vi "Recursive Data Structure for Control Properties.vi"(5 "Max Level (10)":i32, 6 "Draw Controls":T1={"Subpanels"=TRUE, "Tabs"=FALSE, "TypeDefs"=FALSE, "Error Clusters"=enum."Ignore", "DVRs"=enum."Ignore", "Queues & Notifiers"=enum."Ignore"}, 7 "Ignore Image Data (F)":bool, 8 "error in":errorcluster, 9 "Current Level (0)":i32, 10 "Controls[]":refnum<vi>[](array[refnum]), 11 "Parent's name":string) -> (0 "error out":errorcluster, 2 "Results":T3[](array[typedef]))   [LabVIEW 2023, in "VIDoc Parsing.lvlib"]
uses:
  VIDoc Parsing.lvlib
  TypeDefs/Controls Info Cluster.ctl
  <vilib>/picture/picture.llb/imagedata.ctl
  <vilib>/Utility/miscctls.llb/LVKeyTypeDef.ctl
  Settings/Parser Settings/Draw Controls Cluster.ctl
  Settings/Parser Settings/Draw Option Enum.ctl
  <vilib>/Utility/error.llb/Trim Whitespace One-Sided.vi
  Settings/Parser Settings/Parser Settings.lvclass
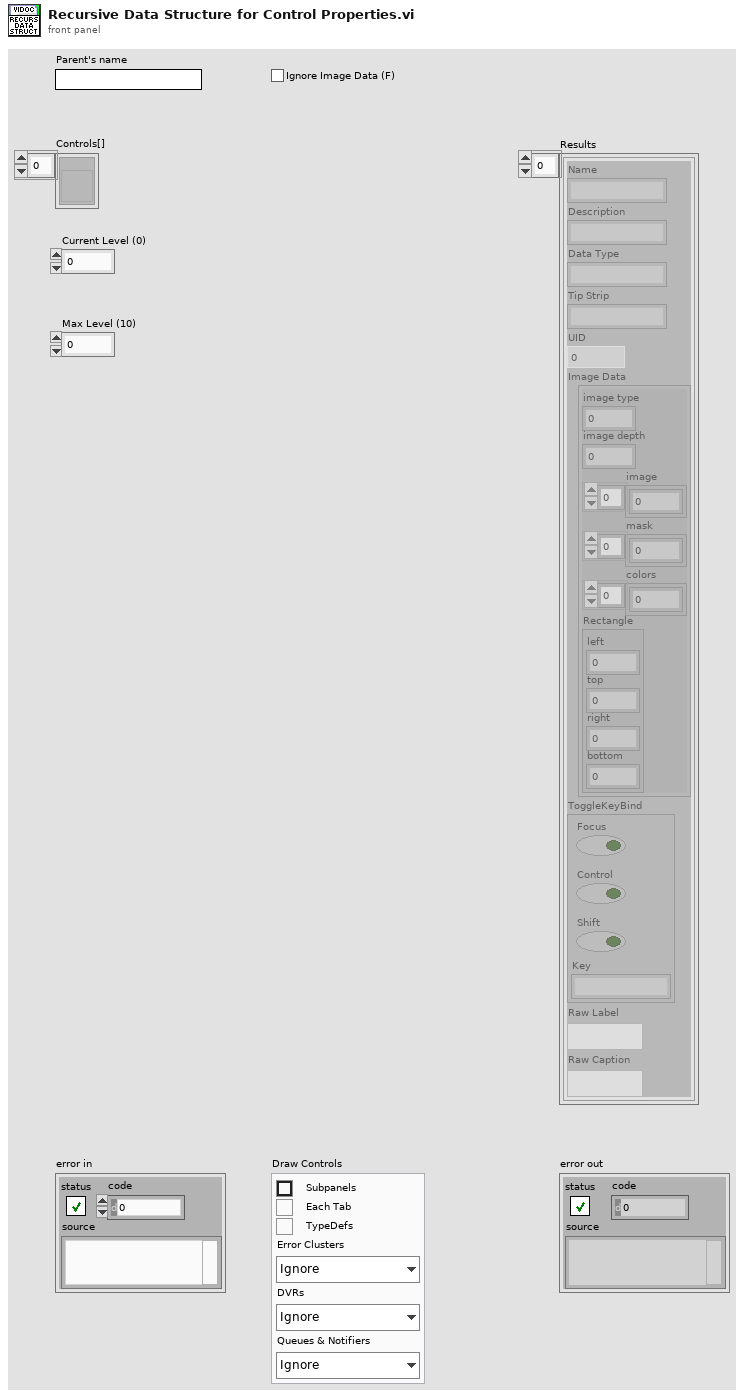
[diagram p1: front panel]
types:
  T1 = typedef "VIDoc Parsing.lvlib/Parser Settings.lvclass/Draw Controls Cluster.ctl" = cluster{"Subpanels":bool, "Tabs":bool, "TypeDefs":bool, "Error Clusters":T2, "DVRs":T2, "Queues & Notifiers":T2}
  T2 = typedef "VIDoc Parsing.lvlib/Parser Settings.lvclass/Draw Option Enum.ctl" = enum16{"Ignore", "Draw", "Draw + Contents"}
  T3 = typedef "VIDoc Parsing.lvlib/Controls Info Cluster.ctl" = cluster{"Name":string, "Description":string, "Data Type":string, "Tip Strip":string, "UID":i32, "Image Data":T4, "ToggleKeyBind":T5, "Raw Label":string, "Raw Caption":string}
  T4 = typedef "imagedata.ctl" = cluster{"image type":i32, "image depth":i32, "image":u8[], "mask":u8[], "colors":u32[], "Rectangle":cluster{"left":i16, "top":i16, "right":i16, "bottom":i16}}
  T5 = typedef "LVKeyTypeDef.ctl" = cluster{"Focus":bool, "Control":bool, "Shift":bool, "Key":string}
  T6 = enum32{"not a typedef", "typedef", "strict typedef", "class private data"}
  T7 = typedef "LVNumericRepresentation.ctl" = enum32{"Extended Precision", "Double Precision", "Single Precision", "Long", "Word", "Byte", "Unsigned Long", "Unsigned Word", "Unsigned Byte", "Complex Extended", "Complex Double", "Complex Single", "Quad", "Unsigned Quad", "Fixed-Point"}
  T8 = typedef "LVStringsAndValuesArrayTypeDef.ctl" = cluster{"String":string, "Value":ext}[]
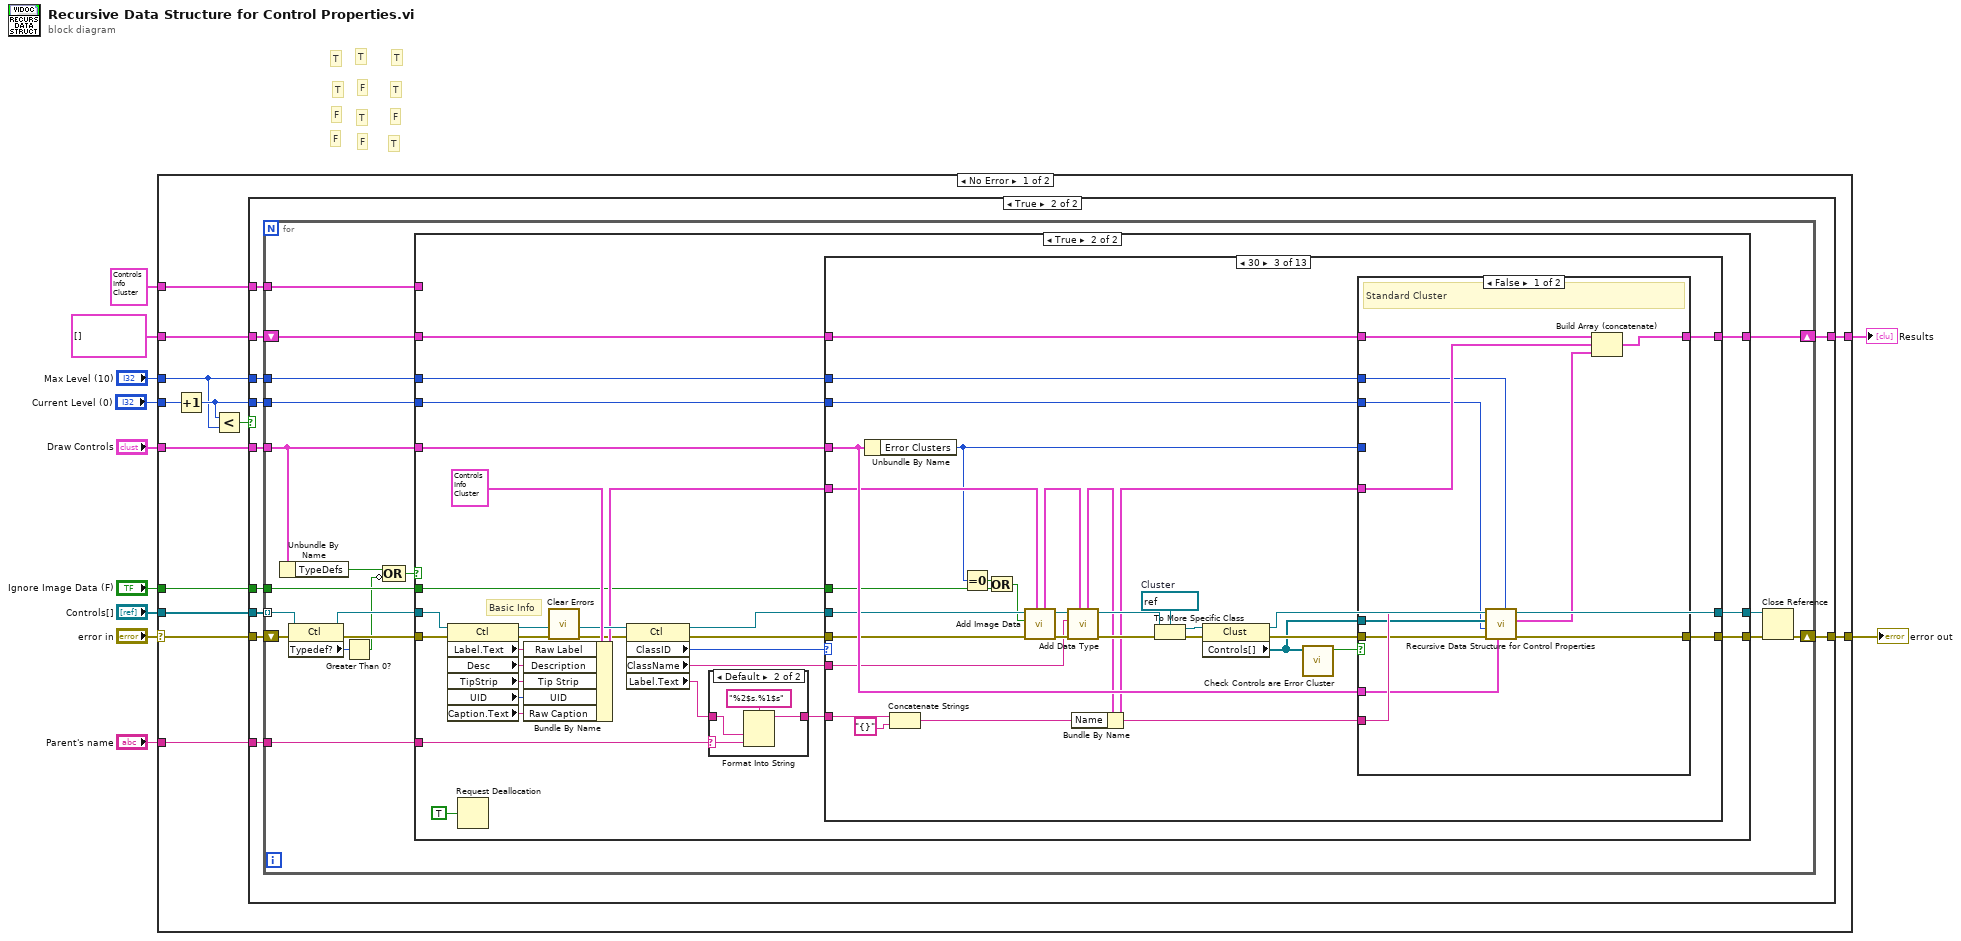
[diagram p0: block diagram]
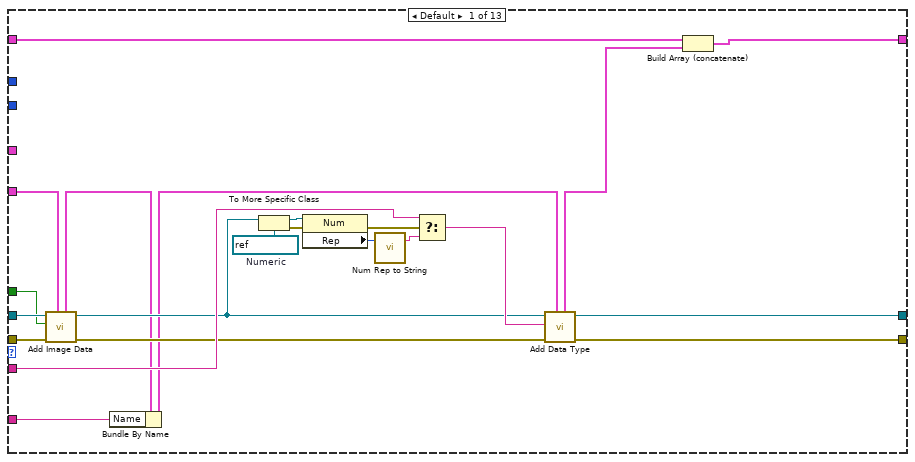
[diagram p5: hidden frame]
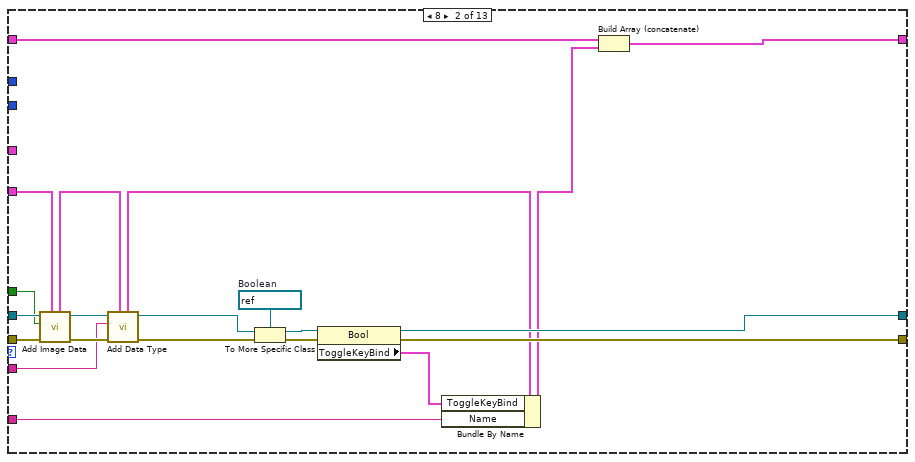
[diagram p6: hidden frame]
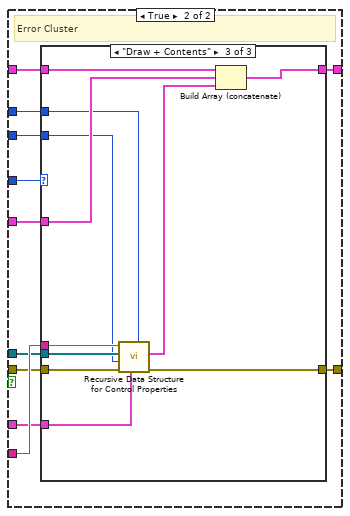
[diagram p7: hidden frame]
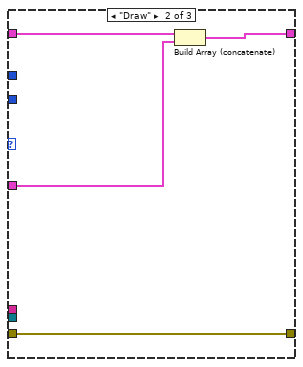
[diagram p9: hidden frame]
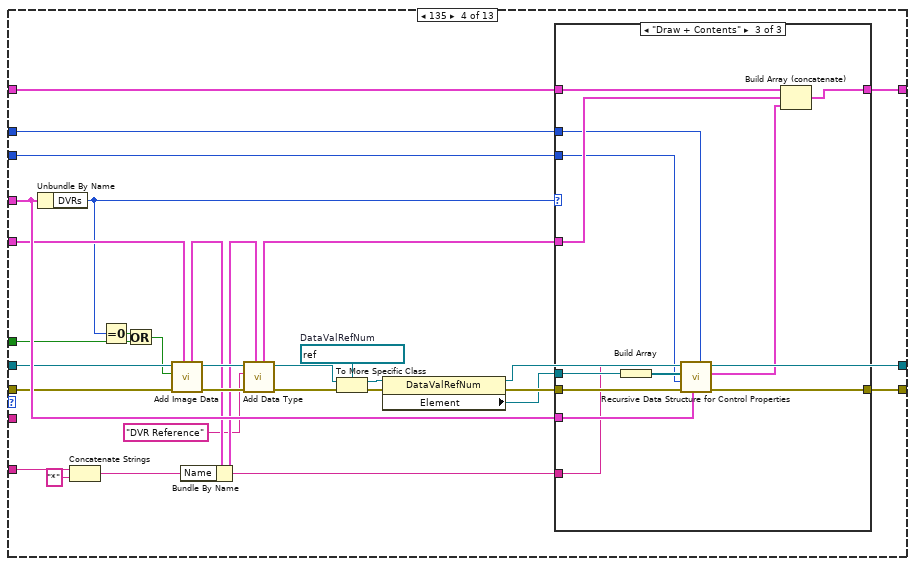
[diagram p10: hidden frame]
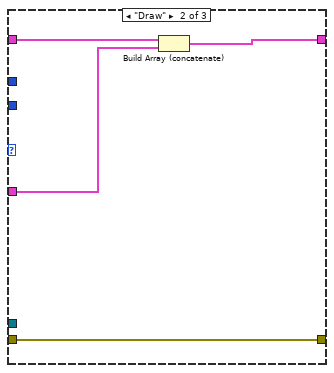
[diagram p12: hidden frame]
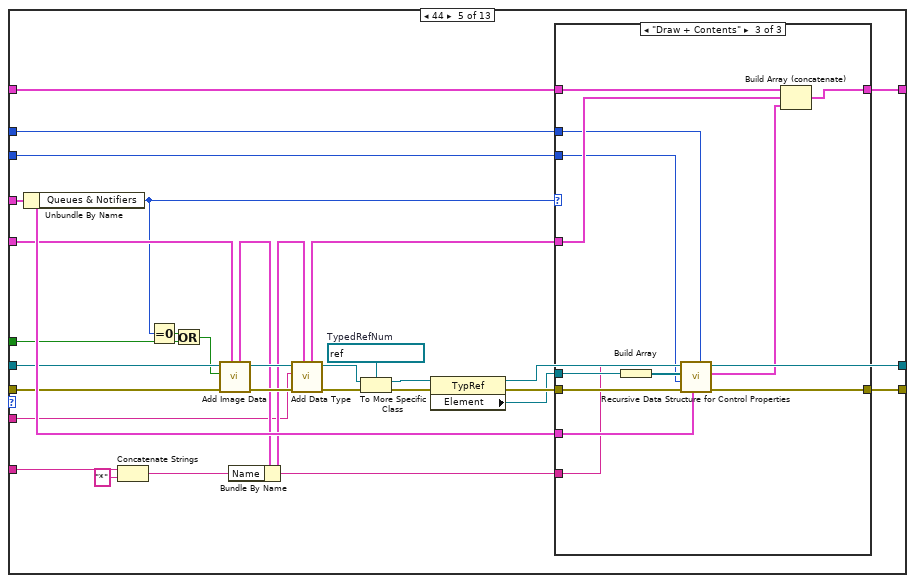
[diagram p13: hidden frame]
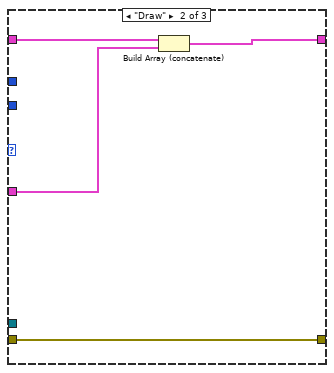
[diagram p15: hidden frame]
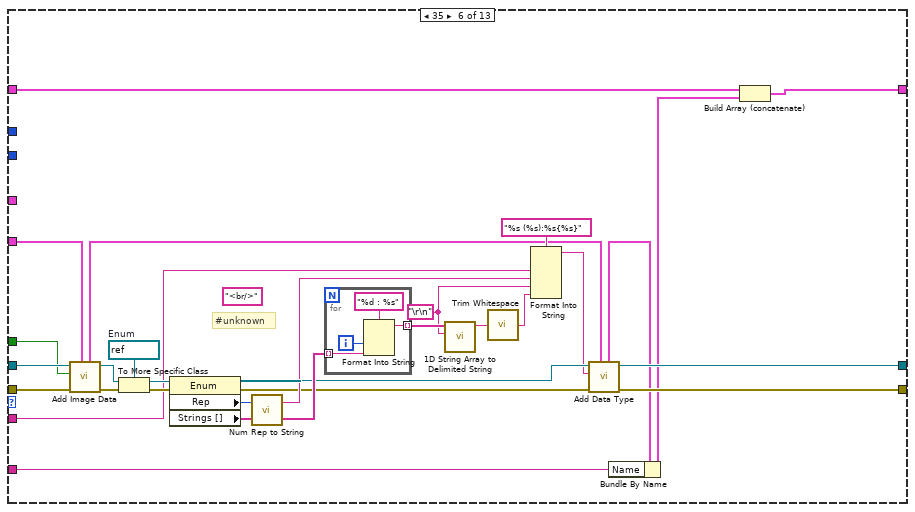
[diagram p16: hidden frame]
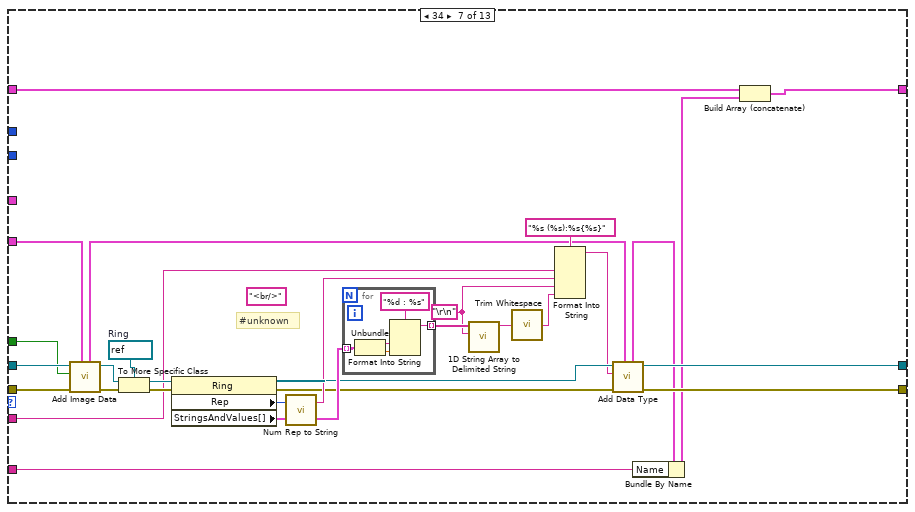
[diagram p17: hidden frame]
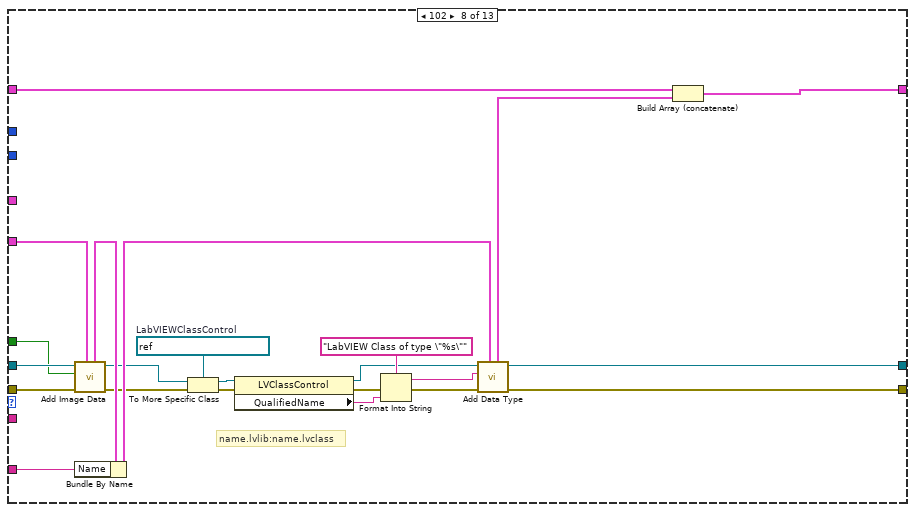
[diagram p18: hidden frame]
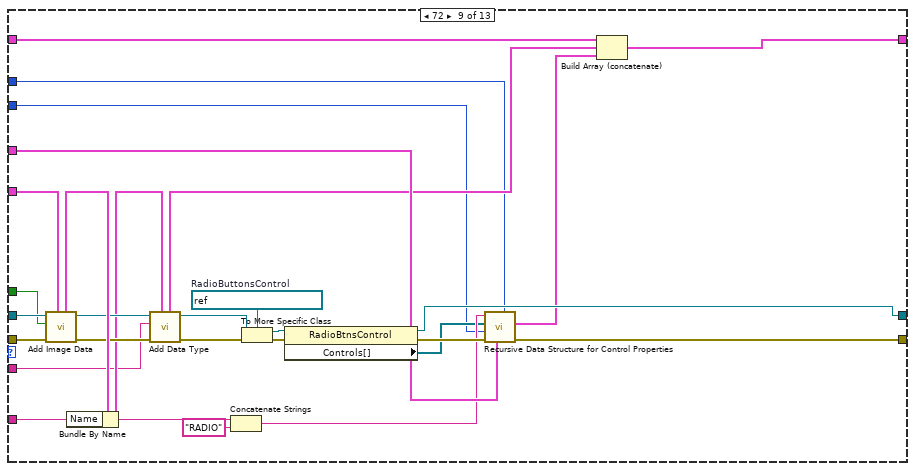
[diagram p19: hidden frame]
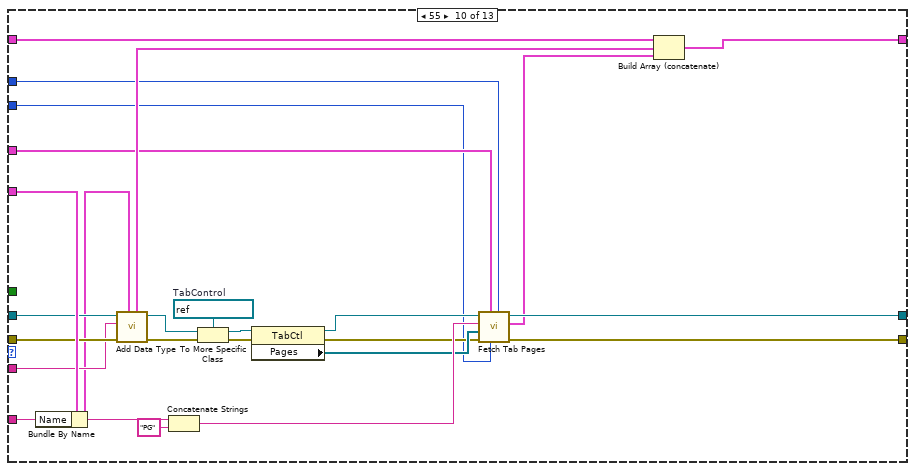
[diagram p20: hidden frame]
diagram:
  # "T"
  # "T"
  # "F"
  # "T"
  # "T"
  # "T"
  # "F"
  # "F"
  # "F"
  # "F"
  # "T"
  # "T"
  n1 = case shown="No Error" "error in" {
    selector: "error in" -> [w20 w517]
    tunnel: "Parent's name" -> [w22 _]
    tunnel: "Controls[]" -> [w24 _]
    tunnel: [w23 w517] -> w9
    tunnel: T3 {"Name"="", "Description"="", "Data Type"="", "Tip Strip"="", "UID"=0, "Image Data"={"image type"=0, "image depth"=0, "image"=[], "mask"=[], "colors"=[], "Rectangle"={"left"=0, "top"=0, "right"=0, "bottom"=0}}, "ToggleKeyBind"={"Focus"=FALSE, "Control"=FALSE, "Shift"=FALSE, "Key"=""}, "Raw Label"="", "Raw Caption"=""} -> [w21 _]
    tunnel: "Draw Controls" -> [w19 _]
    tunnel: "Ignore Image Data (F)" -> [w18 _]
    tunnel: T3[] [] -> [w17 w516]
    tunnel: [w16 w516] -> w3
    tunnel: "Current Level (0)" -> [w15 _]
    tunnel: "Max Level (10)" -> [w13 _]
    frame No Error {
      n2 = Increment(x=w15) -> (x+1=w14:i32)
      n3 = Less?(x=w14, y=w13) -> (x < y?=w12:bool)
      n4 = case shown="True" w12 {
        tunnel: w24 -> [_ w37]
        tunnel: [w25 w36] -> w23
        tunnel: w22 -> [_ w35]
        tunnel: w21 -> [_ w34]
        tunnel: w20 -> [w25 w33]
        tunnel: w19 -> [_ w32]
        tunnel: w18 -> [_ w31]
        tunnel: w17 -> [w26 w30]
        tunnel: [w26 w29] -> w16
        tunnel: w14 -> [_ w28]
        tunnel: w13 -> [_ w27]
        frame False {
        }
        frame True {
          n5 = for {
            tunnel: w37 -> [w48] mode=indexing
            tunnel: w35 -> [w56]
            tunnel: w34 -> [w55]
            shift-right: [w44] -> w36
            shift-left: w33 -> [w51]
            tunnel: w32 -> [w54]
            tunnel: w31 -> [w53]
            shift-right: [w46] -> w29
            shift-left: w30 -> [w52]
            tunnel: w28 -> [w39]
            tunnel: w27 -> [w38]
            n6 = Unbundle By Name(w54) -> ("TypeDefs"=w42:bool)
            n7 = property class="Ctl"(reference=w48, error in=w51) -> (reference out=w49:refnum<vi>, error out=w50:errorcluster, "Typedef?"=w47:T6)
            n8 = Greater Than 0?(x=w47) -> (x > 0?=w41:bool)
            n9 = Compound Arithmetic op=OR(w42, invert w41) -> (w40:bool)
            n10 = case shown="True" w40 {
              tunnel: w56 -> [_ w87]
              tunnel: w55 -> [_ _]
              tunnel: [w58 w64] -> w45
              tunnel: w54 -> [_ w79]
              tunnel: w53 -> [_ w69]
              tunnel: w52 -> [w59 w68]
              tunnel: w50 -> [w58 w67]
              tunnel: w49 -> [w57 w66]
              tunnel: [w59 w63] -> w46
              tunnel: [w57 w65] -> w43
              tunnel: w39 -> [_ w61]
              tunnel: w38 -> [_ w60]
              frame False {
                # "Is TypeDef but options say not to process"
              }
              frame True {
                # "Basic Info"
                n11 = property class="Ctl"(reference=w66, error in=w67) -> (reference out=w71:refnum<vi>, error out=w72:errorcluster, "Label.Text"=w77:string, "Desc"=w76:string, "TipStrip"=w75:string, "UID"=w74:i32, "Caption.Text"=w73:string)
                n12 = Request Deallocation(TRUE ("flag")) -> ()
                n13 = Bundle By Name(cluster=T3 {"Name"="", "Description"="", "Data Type"="", "Tip Strip"="", "UID"=0, "Image Data"={"image type"=0, "image depth"=0, "image"=[], "mask"=[], "colors"=[], "Rectangle"={"left"=0, "top"=0, "right"=0, "bottom"=0}}, "ToggleKeyBind"={"Focus"=FALSE, "Control"=FALSE, "Shift"=FALSE, "Key"=""}, "Raw Label"="", "Raw Caption"=""}, "Raw Label"=w77, "Description"=w76, "Tip Strip"=w75, "UID"=w74, "Raw Caption"=w73) -> (w70:T3)
                n14 = call <vilib>:"Clear Errors.vi"("error in (no error)"=w72) -> ("error out"=w62:errorcluster)  [unwired: 5 in, 1 out]
                n15 = property class="Ctl"(reference=w71, error in=w62) -> (reference out=w81:refnum<vi>, error out=w80:errorcluster, "ClassID"=w84:u32, "ClassName"=w85:string, "Label.Text"=w83:string)
                n16 = case shown="Default" w87 {
                  selector: w87 -> [_ w90]
                  tunnel: w83 -> [w88 w91]
                  tunnel: [w88 w89] -> w86
                  frame "" {
                  }
                  frame Default {
                    n17 = Format Into String(format string="%2$s.%1$s", w91, w90) -> (resulting string=w89:string)  [unwired: 2 in, 1 out]
                  }
                }
                n18 = case shown="30" w84 {
                  tunnel: w81 -> [w106 w130 w154 w225 w274 w322 w355 w385 w414 w437 w461 w487 w514]
                  tunnel: [w100 w131 w164 w229 w278 w308 w341 w370 w401 w424 w449 w477 w504] -> w64
                  tunnel: w86 -> [w105 w126 w161 w234 w282 w303 w336 w380 w409 w439 w456 w493 w507]
                  tunnel: [w98 w132 w160 w228 w277 w307 w340 w373 w415 w428 w451 w479 w498] -> w65
                  tunnel: w85 -> [w109 w120 w146 _ w256 w325 w358 _ w404 w435 _ w490 w503]
                  tunnel: w80 -> [w107 w129 w155 w224 w273 w321 w354 w384 w413 w436 w460 w486 w513]
                  tunnel: w79 -> [_ _ w158 w226 w275 _ _ _ w400 w423 _ w476 w515]
                  tunnel: w70 -> [w104 w127 w153 w223 w272 w319 w352 w382 w411 w440 w458 w484 w509]
                  tunnel: w69 -> [w103 w128 w139 w208 w258 w320 w353 w383 w412 _ w459 w485 w512]
                  tunnel: w68 -> [w95 w125 w142 w211 w261 w315 w348 w378 w397 w432 w447 w471 w501]
                  tunnel: [w94 w124 w141 w209 w259 w314 w347 w377 w396 w431 w446 w470 w500] -> w63
                  tunnel: w61 -> [_ _ w136 w206 w255 _ _ _ w392 w420 _ w466 _]
                  tunnel: w60 -> [_ _ w137 w207 w254 _ _ _ w393 w421 _ w467 _]
                  frame Default {
                    w111 = refnum<vi> refnum  # Numeric
                    n19 = call "Add Image Data.vi"("Control Info Cluster in"=w104, "error in (no error)"=w107, "Ignore Image Data"=w103, "Control in"=w106) -> ("error out"=w101:errorcluster, "Control out"=w99:refnum<vi>, "Control Info Cluster out"=w97:T3)  [unwired: 5 in]
                    n20 = Bundle By Name(cluster=w97, "Name"=w105) -> (w96:T3)
                    n21 = To More Specific Class(target class=w111, reference=w99) -> (specific class reference=w112:refnum<vi>, error out=w113:errorcluster)  [unwired: 1 in]
                    n22 = property class="Num"(reference=w112, error in=w113) -> (error out=w110:errorcluster, "Rep"=w114:T7)  [unwired: 1 out]
                    n23 = call "Num Rep to String.vi"("Rep"=w114) -> ("String"=w108:string)  [unwired: 2 in]
                    n24 = Select(t=w109, s=w110, f=w108) -> (s? t:f=w102:string)
                    n25 = call "Add Data Type.vi"("Control Info Cluster in"=w96, "error in (no error)"=w101, "Data Type String"=w102, "Control in"=w99) -> ("error out"=w100:errorcluster, "Control out"=w98:refnum<vi>, "Control Info Cluster out"=w93:T3)  [unwired: 4 in, 1 out]
                    n26 = Build Array (concatenate)(w95, w93) -> (w94:T3[])
                  }
                  frame 8 {
                    w135 = refnum<vi> refnum  # Boolean
                    n27 = call "Add Image Data.vi"("Control Info Cluster in"=w127, "error in (no error)"=w129, "Ignore Image Data"=w128, "Control in"=w130) -> ("error out"=w121:errorcluster, "Control out"=w123:refnum<vi>, "Control Info Cluster out"=w117:T3)  [unwired: 5 in]
                    n28 = call "Add Data Type.vi"("Control Info Cluster in"=w117, "error in (no error)"=w121, "Data Type String"=w120, "Control in"=w123) -> ("error out"=w118:errorcluster, "Control out"=w122:refnum<vi>, "Control Info Cluster out"=w116:T3)  [unwired: 4 in, 1 out]
                    n29 = To More Specific Class(target class=w135, reference=w122, error in=w118) -> (specific class reference=w134:refnum<vi>, error out=w133:errorcluster)
                    n30 = property class="Bool"(reference=w134, error in=w133) -> (reference out=w132:refnum<vi>, error out=w131:errorcluster, "ToggleKeyBind"=w119:T5)
                    n31 = Bundle By Name(cluster=w116, "ToggleKeyBind"=w119, "Name"=w126) -> (w115:T3)
                    n32 = Build Array (concatenate)(w125, w115) -> (w124:T3[])
                  }
                  frame 30 {
                    w166 = refnum<vi> refnum  # Cluster
                    n33 = Unbundle By Name(w158) -> ("Error Clusters"=w152:T2)
                    n34 = Concatenate Strings(w161, "{}" ("string")) -> (w143:string)
                    n35 = Equal To 0?(x=w152) -> (x = 0?=w151:bool)
                    n36 = Or(x=w151, y=w139) -> (x .or. y?=w140:bool)
                    n37 = call "Add Image Data.vi"("Control Info Cluster in"=w153, "error in (no error)"=w155, "Ignore Image Data"=w140, "Control in"=w154) -> ("error out"=w150:errorcluster, "Control out"=w148:refnum<vi>, "Control Info Cluster out"=w145:T3)  [unwired: 5 in]
                    n38 = call "Add Data Type.vi"("Control Info Cluster in"=w145, "error in (no error)"=w150, "Data Type String"=w146, "Control in"=w148) -> ("error out"=w149:errorcluster, "Control out"=w147:refnum<vi>, "Control Info Cluster out"=w144:T3)  [unwired: 4 in, 1 out]
                    n39 = Bundle By Name(cluster=w144, "Name"=w143) -> (w138:T3)
                    n40 = To More Specific Class(target class=w166, reference=w147, error in=w149) -> (specific class reference=w165:refnum<vi>, error out=w163:errorcluster)
                    n41 = property class="Clust"(reference=w165, error in=w163) -> (reference out=w160:refnum<vi>, error out=w159:errorcluster, "Controls[]"=w157:refnum<vi>[])
                    n42 = call "Check Controls are Error Cluster.vi"("Controls[]"=w157) -> ("Error Cluster"=w156:bool)  [unwired: 10 in]
                    n43 = case shown="False" w156 {
                      tunnel: [w174 w188] -> w164
                      tunnel: w143 -> [w177 w187]
                      tunnel: w157 -> [w173 w186]
                      tunnel: w159 -> [w176 w185]
                      tunnel: w158 -> [w175 w184]
                      tunnel: w152 -> [_ w183]
                      tunnel: w142 -> [w172 w180]
                      tunnel: [w171 w181] -> w141
                      tunnel: w138 -> [w169 w182]
                      tunnel: w137 -> [w168 w179]
                      tunnel: w136 -> [w167 w178]
                      frame False {
                        # "Standard Cluster"
                        n44 = call "Recursive Data Structure for Control Properties.vi"("Max Level (10)"=w168, "Draw Controls"=w175, "error in"=w176, "Current Level (0)"=w167, "Controls[]"=w173, "Parent's name"=w177) -> ("error out"=w174:errorcluster, "Results"=w170:T3[])  [unwired: 4 in]
                        n45 = Build Array (concatenate)(w172, w169, w170) -> (w171:T3[])
                      }
                      frame True {
                        # "Error Cluster"
                        n46 = case shown="\"Draw + Contents\"" w183 {
                          tunnel: w186 -> [_ _ w201]
                          tunnel: [w190 w194 w204] -> w188
                          tunnel: w187 -> [_ _ w202]
                          tunnel: w185 -> [w190 w194 w205]
                          tunnel: w184 -> [_ _ w203]
                          tunnel: w182 -> [_ w191 w198]
                          tunnel: [w189 w192 w199] -> w181
                          tunnel: w180 -> [w189 w193 w200]
                          tunnel: w179 -> [_ _ w196]
                          tunnel: w178 -> [_ _ w195]
                          frame "Ignore" {
                          }
                          frame "Draw" {
                            n47 = Build Array (concatenate)(w193, w191) -> (w192:T3[])
                          }
                          frame "Draw + Contents" {
                            n48 = call "Recursive Data Structure for Control Properties.vi"("Max Level (10)"=w196, "Draw Controls"=w203, "error in"=w205, "Current Level (0)"=w195, "Controls[]"=w201, "Parent's name"=w202) -> ("error out"=w204:errorcluster, "Results"=w197:T3[])  [unwired: 4 in]
                            n49 = Build Array (concatenate)(w200, w198, w197) -> (w199:T3[])
                          }
                        }
                      }
                    }
                  }
                  frame 135 {
                    w233 = refnum<vi> refnum  # DataValRefNum
                    n50 = Unbundle By Name(w226) -> ("DVRs"=w221:T2)
                    n51 = Concatenate Strings(w234, "*" ("string")) -> (w214:string)
                    n52 = Equal To 0?(x=w221) -> (x = 0?=w222:bool)
                    n53 = Or(x=w222, y=w208) -> (x .or. y?=w220:bool)
                    n54 = call "Add Image Data.vi"("Control Info Cluster in"=w223, "error in (no error)"=w224, "Ignore Image Data"=w220, "Control in"=w225) -> ("error out"=w218:errorcluster, "Control out"=w219:refnum<vi>, "Control Info Cluster out"=w215:T3)  [unwired: 5 in]
                    n55 = Bundle By Name(cluster=w215, "Name"=w214) -> (w213:T3)
                    n56 = call "Add Data Type.vi"("Control Info Cluster in"=w213, "error in (no error)"=w218, "Data Type String"="DVR Reference" ("input 2"), "Control in"=w219) -> ("error out"=w217:errorcluster, "Control out"=w216:refnum<vi>, "Control Info Cluster out"=w210:T3)  [unwired: 4 in, 1 out]
                    n57 = To More Specific Class(target class=w233, reference=w216, error in=w217) -> (specific class reference=w227:refnum<vi>, error out=w232:errorcluster)
                    n58 = property class="DataValRefNum"(reference=w227, error in=w232) -> (reference out=w228:refnum<vi>, error out=w231:errorcluster, "Element"=w230:refnum<vi>)
                    n59 = case shown="\"Draw + Contents\"" w221 {
                      tunnel: w214 -> [_ _ w246]
                      tunnel: w231 -> [w237 w241 w249]
                      tunnel: w230 -> [_ _ w253]
                      tunnel: [w237 w241 w248] -> w229
                      tunnel: w226 -> [_ _ w247]
                      tunnel: w211 -> [w236 w240 w252]
                      tunnel: w210 -> [_ w238 w250]
                      tunnel: [w236 w239 w251] -> w209
                      tunnel: w207 -> [_ _ w243]
                      tunnel: w206 -> [_ _ w242]
                      frame "Ignore" {
                      }
                      frame "Draw" {
                        n60 = Build Array (concatenate)(w240, w238) -> (w239:T3[])
                      }
                      frame "Draw + Contents" {
                        n61 = Build Array(w253) -> (w245:refnum<vi>[])
                        n62 = call "Recursive Data Structure for Control Properties.vi"("Max Level (10)"=w243, "Draw Controls"=w247, "error in"=w249, "Current Level (0)"=w242, "Controls[]"=w245, "Parent's name"=w246) -> ("error out"=w248:errorcluster, "Results"=w244:T3[])  [unwired: 4 in]
                        n63 = Build Array (concatenate)(w252, w250, w244) -> (w251:T3[])
                      }
                    }
                  }
                  frame 44 {
                    w257 = refnum<vi> refnum  # TypedRefNum
                    n64 = Unbundle By Name(w275) -> ("Queues & Notifiers"=w270:T2)
                    n65 = Concatenate Strings(w282, "*" ("string")) -> (w263:string)
                    n66 = Equal To 0?(x=w270) -> (x = 0?=w271:bool)
                    n67 = Or(x=w271, y=w258) -> (x .or. y?=w269:bool)
                    n68 = call "Add Image Data.vi"("Control Info Cluster in"=w272, "error in (no error)"=w273, "Ignore Image Data"=w269, "Control in"=w274) -> ("error out"=w267:errorcluster, "Control out"=w268:refnum<vi>, "Control Info Cluster out"=w264:T3)  [unwired: 5 in]
                    n69 = Bundle By Name(cluster=w264, "Name"=w263) -> (w262:T3)
                    n70 = call "Add Data Type.vi"("Control Info Cluster in"=w262, "error in (no error)"=w267, "Data Type String"=w256, "Control in"=w268) -> ("error out"=w266:errorcluster, "Control out"=w265:refnum<vi>, "Control Info Cluster out"=w260:T3)  [unwired: 4 in, 1 out]
                    n71 = To More Specific Class(target class=w257, reference=w265, error in=w266) -> (specific class reference=w276:refnum<vi>, error out=w281:errorcluster)
                    n72 = property class="TypRef"(reference=w276, error in=w281) -> (reference out=w277:refnum<vi>, error out=w280:errorcluster, "Element"=w279:refnum<vi>)
                    n73 = case shown="\"Draw + Contents\"" w270 {
                      tunnel: w263 -> [_ _ w294]
                      tunnel: w280 -> [w285 w289 w297]
                      tunnel: w279 -> [_ _ w301]
                      tunnel: [w285 w289 w296] -> w278
                      tunnel: w275 -> [_ _ w295]
                      tunnel: w261 -> [w284 w288 w300]
                      tunnel: w260 -> [_ w286 w298]
                      tunnel: [w284 w287 w299] -> w259
                      tunnel: w255 -> [_ _ w291]
                      tunnel: w254 -> [_ _ w290]
                      frame "Ignore" {
                      }
                      frame "Draw" {
                        n74 = Build Array (concatenate)(w288, w286) -> (w287:T3[])
                      }
                      frame "Draw + Contents" {
                        n75 = Build Array(w301) -> (w293:refnum<vi>[])
                        n76 = call "Recursive Data Structure for Control Properties.vi"("Max Level (10)"=w290, "Draw Controls"=w295, "error in"=w297, "Current Level (0)"=w291, "Controls[]"=w293, "Parent's name"=w294) -> ("error out"=w296:errorcluster, "Results"=w292:T3[])  [unwired: 4 in]
                        n77 = Build Array (concatenate)(w300, w298, w292) -> (w299:T3[])
                      }
                    }
                  }
                  frame 35 {
                    w311 = "\r\n"
                    (unwired) "<br/>" ("string")
                    w330 = refnum<vi> refnum  # Enum
                    # "#unknown"
                    n78 = call "Add Image Data.vi"("Control Info Cluster in"=w319, "error in (no error)"=w321, "Ignore Image Data"=w320, "Control in"=w322) -> ("error out"=w318:errorcluster, "Control out"=w323:refnum<vi>, "Control Info Cluster out"=w305:T3)  [unwired: 5 in]
                    n79 = To More Specific Class(target class=w330, reference=w323, error in=w318) -> (specific class reference=w329:refnum<vi>, error out=w328:errorcluster)
                    n80 = property class="Enum"(reference=w329, error in=w328) -> (reference out=w310:refnum<vi>, error out=w309:errorcluster, "Rep"=w317:T7, "Strings []"=w327:string[])
                    n81 = call "Num Rep to String.vi"("Rep"=w317) -> ("String"=w316:string)  [unwired: 2 in]
                    n82 = for {
                      tunnel: w327 -> [w332] mode=indexing
                      tunnel: [w333] -> w313 mode=indexing
                      i -> [w334]
                      n83 = Format Into String(format string="%d : %s", w334, w332) -> (resulting string=w333:string)  [unwired: 2 in, 1 out]
                    }
                    n84 = call <vilib>:"1D String Array to Delimited String.vi"("delimiter"=w311, "string array"=w313) -> ("delimited string"=w312:string)  [unwired: 9 in]
                    n85 = call <vilib>:"Trim Whitespace.vi"("string"=w312) -> ("trimmed string"=w324:string)  [unwired: 1 in]
                    n86 = Format Into String(format string="%s (%s):%s{%s}", w325, w316, w311, w324) -> (resulting string=w306:string)  [unwired: 2 in, 1 out]
                    n87 = call "Add Data Type.vi"("Control Info Cluster in"=w305, "error in (no error)"=w309, "Data Type String"=w306, "Control in"=w310) -> ("error out"=w308:errorcluster, "Control out"=w307:refnum<vi>, "Control Info Cluster out"=w304:T3)  [unwired: 4 in, 1 out]
                    n88 = Bundle By Name(cluster=w304, "Name"=w303) -> (w302:T3)
                    n89 = Build Array (concatenate)(w315, w302) -> (w314:T3[])
                  }
                  frame 34 {
                    w344 = "\r\n"
                    (unwired) "<br/>" ("string")
                    w363 = refnum<vi> refnum  # Ring
                    # "#unknown"
                    n90 = call "Add Image Data.vi"("Control Info Cluster in"=w352, "error in (no error)"=w354, "Ignore Image Data"=w353, "Control in"=w355) -> ("error out"=w351:errorcluster, "Control out"=w356:refnum<vi>, "Control Info Cluster out"=w338:T3)  [unwired: 5 in]
                    n91 = To More Specific Class(target class=w363, reference=w356, error in=w351) -> (specific class reference=w362:refnum<vi>, error out=w361:errorcluster)
                    n92 = property class="Ring"(reference=w362, error in=w361) -> (reference out=w343:refnum<vi>, error out=w342:errorcluster, "Rep"=w350:T7, "StringsAndValues[]"=w360:T8)
                    n93 = call "Num Rep to String.vi"("Rep"=w350) -> ("String"=w349:string)  [unwired: 2 in]
                    n94 = for {
                      tunnel: w360 -> [w366] mode=indexing
                      tunnel: [w368] -> w346 mode=indexing
                      n95 = Unbundle(w366) -> ("String"=w364:string, "Value"=w365:ext)
                      n96 = Format Into String(format string="%d : %s", w365, w364) -> (resulting string=w368:string)  [unwired: 2 in, 1 out]
                    }
                    n97 = call <vilib>:"1D String Array to Delimited String.vi"("delimiter"=w344, "string array"=w346) -> ("delimited string"=w345:string)  [unwired: 9 in]
                    n98 = call <vilib>:"Trim Whitespace.vi"("string"=w345) -> ("trimmed string"=w357:string)  [unwired: 1 in]
                    n99 = Format Into String(format string="%s (%s):%s{%s}", w358, w349, w344, w357) -> (resulting string=w339:string)  [unwired: 2 in, 1 out]
                    n100 = call "Add Data Type.vi"("Control Info Cluster in"=w338, "error in (no error)"=w342, "Data Type String"=w339, "Control in"=w343) -> ("error out"=w341:errorcluster, "Control out"=w340:refnum<vi>, "Control Info Cluster out"=w337:T3)  [unwired: 4 in, 1 out]
                    n101 = Bundle By Name(cluster=w337, "Name"=w336) -> (w335:T3)
                    n102 = Build Array (concatenate)(w348, w335) -> (w347:T3[])
                  }
                  frame 102 {
                    w390 = refnum<vi> refnum  # LabVIEWClassControl
                    # "name.lvlib:name.lvclass"
                    n103 = call "Add Image Data.vi"("Control Info Cluster in"=w382, "error in (no error)"=w384, "Ignore Image Data"=w383, "Control in"=w385) -> ("error out"=w376:errorcluster, "Control out"=w375:refnum<vi>, "Control Info Cluster out"=w381:T3)  [unwired: 5 in]
                    n104 = Bundle By Name(cluster=w381, "Name"=w380) -> (w379:T3)
                    n105 = To More Specific Class(target class=w390, reference=w375, error in=w376) -> (specific class reference=w389:refnum<vi>, error out=w388:errorcluster)
                    n106 = property class="LVClassControl"(reference=w389, error in=w388) -> (reference out=w374:refnum<vi>, error out=w387:errorcluster, "QualifiedName"=w386:string)
                    n107 = Format Into String(format string="LabVIEW Class of type \"%s\"", error in=w387, w386) -> (resulting string=w372:string, error out=w371:errorcluster)  [unwired: 1 in]
                    n108 = call "Add Data Type.vi"("Control Info Cluster in"=w379, "error in (no error)"=w371, "Data Type String"=w372, "Control in"=w374) -> ("error out"=w370:errorcluster, "Control out"=w373:refnum<vi>, "Control Info Cluster out"=w369:T3)  [unwired: 4 in, 1 out]
                    n109 = Build Array (concatenate)(w378, w369) -> (w377:T3[])
                  }
                  frame 72 {
                    w419 = refnum<vi> refnum  # RadioButtonsControl
                    n110 = call "Add Image Data.vi"("Control Info Cluster in"=w411, "error in (no error)"=w413, "Ignore Image Data"=w412, "Control in"=w414) -> ("error out"=w406:errorcluster, "Control out"=w408:refnum<vi>, "Control Info Cluster out"=w410:T3)  [unwired: 5 in]
                    n111 = Bundle By Name(cluster=w410, "Name"=w409) -> (w405:T3)
                    n112 = call "Add Data Type.vi"("Control Info Cluster in"=w405, "error in (no error)"=w406, "Data Type String"=w404, "Control in"=w408) -> ("error out"=w403:errorcluster, "Control out"=w407:refnum<vi>, "Control Info Cluster out"=w395:T3)  [unwired: 4 in, 1 out]
                    n113 = Concatenate Strings(w409, "RADIO" ("string")) -> (w399:string)
                    n114 = To More Specific Class(target class=w419, reference=w407, error in=w403) -> (specific class reference=w418:refnum<vi>, error out=w417:errorcluster)
                    n115 = property class="RadioBtnsControl"(reference=w418, error in=w417) -> (reference out=w415:refnum<vi>, error out=w402:errorcluster, "Controls[]"=w398:refnum<vi>[])
                    n116 = call "Recursive Data Structure for Control Properties.vi"("Max Level (10)"=w393, "Draw Controls"=w400, "error in"=w402, "Current Level (0)"=w392, "Controls[]"=w398, "Parent's name"=w399) -> ("error out"=w401:errorcluster, "Results"=w394:T3[])  [unwired: 4 in]
                    n117 = Build Array (concatenate)(w397, w395, w394) -> (w396:T3[])
                  }
                  frame 55 {
                    w444 = refnum<vi> refnum  # TabControl
                    n118 = Bundle By Name(cluster=w440, "Name"=w439) -> (w434:T3)
                    n119 = call "Add Data Type.vi"("Control Info Cluster in"=w434, "error in (no error)"=w436, "Data Type String"=w435, "Control in"=w437) -> ("error out"=w433:errorcluster, "Control out"=w438:refnum<vi>, "Control Info Cluster out"=w430:T3)  [unwired: 4 in, 1 out]
                    n120 = Concatenate Strings(w439, "PG" ("string")) -> (w427:string)
                    n121 = To More Specific Class(target class=w444, reference=w438, error in=w433) -> (specific class reference=w443:refnum<vi>, error out=w442:errorcluster)
                    n122 = property class="TabCtl"(reference=w443, error in=w442) -> (reference out=w429:refnum<vi>, error out=w425:errorcluster, "Pages"=w426:refnum<vi>[])
                    n123 = call "Fetch Tab Pages.vi"("Max Level (10)"=w421, "Current Level (0)"=w420, "Draw Controls"=w423, "error in (no error)"=w425, "Pages"=w426, "Parent"=w427, "Tab Ref in"=w429) -> ("error out"=w424:errorcluster, "Results"=w422:T3[], "Tab Ref out"=w428:refnum<vi>)  [unwired: 2 in]
                    n124 = Build Array (concatenate)(w432, w430, w422) -> (w431:T3[])
                  }
                  frame 18 {
                    w465 = refnum<vi> refnum  # Digital
                    n125 = call "Add Image Data.vi"("Control Info Cluster in"=w458, "error in (no error)"=w460, "Ignore Image Data"=w459, "Control in"=w461) -> ("error out"=w455:errorcluster, "Control out"=w462:refnum<vi>, "Control Info Cluster out"=w457:T3)  [unwired: 5 in]
                    n126 = Bundle By Name(cluster=w457, "Name"=w456) -> (w448:T3)
                    n127 = To More Specific Class(target class=w465, reference=w462, error in=w455) -> (specific class reference=w464:refnum<vi>, error out=w463:errorcluster)
                    n128 = property class="DigNum"(reference=w464, error in=w463) -> (reference out=w452:refnum<vi>, error out=w450:errorcluster, "Rep"=w454:T7)
                    n129 = call "Num Rep to String.vi"("Rep"=w454) -> ("String"=w453:string)  [unwired: 2 in]
                    n130 = call "Add Data Type.vi"("Control Info Cluster in"=w448, "error in (no error)"=w450, "Data Type String"=w453, "Control in"=w452) -> ("error out"=w449:errorcluster, "Control out"=w451:refnum<vi>, "Control Info Cluster out"=w445:T3)  [unwired: 4 in, 1 out]
                    n131 = Build Array (concatenate)(w447, w445) -> (w446:T3[])
                  }
                  frame 14 {
                    w497 = refnum<vi> refnum  # Array
                    n132 = call "Add Image Data.vi"("Control Info Cluster in"=w484, "error in (no error)"=w486, "Ignore Image Data"=w485, "Control in"=w487) -> ("error out"=w482:errorcluster, "Control out"=w488:refnum<vi>, "Control Info Cluster out"=w483:T3)  [unwired: 5 in]
                    n133 = Concatenate Strings(w493, "[]" ("string")) -> (w474:string)
                    n134 = Bundle By Name(cluster=w483, "Name"=w474) -> (w472:T3)
                    n135 = To More Specific Class(target class=w497, reference=w488, error in=w482) -> (specific class reference=w496:refnum<vi>, error out=w494:errorcluster)
                    n136 = property class="Arr"(reference=w496, error in=w494) -> (reference out=w481:refnum<vi>, error out=w480:errorcluster, "Array Element"=w495:refnum<vi>, "NumDims"=w489:u32)
                    n137 = Build Array(w495) -> (w475:refnum<vi>[])
                    n138 = Format Into String(format string="%2$d Dimensional %1$s", w490, w489) -> (resulting string=w473:string)  [unwired: 2 in, 1 out]
                    n139 = call "Add Data Type.vi"("Control Info Cluster in"=w472, "error in (no error)"=w480, "Data Type String"=w473, "Control in"=w481) -> ("error out"=w478:errorcluster, "Control out"=w479:refnum<vi>, "Control Info Cluster out"=w469:T3)  [unwired: 4 in, 1 out]
                    n140 = call "Recursive Data Structure for Control Properties.vi"("Max Level (10)"=w467, "Draw Controls"=w476, "error in"=w478, "Current Level (0)"=w466, "Controls[]"=w475, "Parent's name"=w474) -> ("error out"=w477:errorcluster, "Results"=w468:T3[])  [unwired: 4 in]
                    n141 = Build Array (concatenate)(w471, w469, w468) -> (w470:T3[])
                  }
                  frame 65 {
                    (unwired) refnum<vi> refnum ("Sub Panel")
                    n142 = Unbundle By Name(w515) -> ("Subpanels"=w510:bool)
                    n143 = Compound Arithmetic op=OR(invert w510, w512) -> (w511:bool)
                    n144 = call "Add Image Data.vi"("Control Info Cluster in"=w509, "error in (no error)"=w513, "Ignore Image Data"=w511, "Control in"=w514) -> ("error out"=w506:errorcluster, "Control out"=w505:refnum<vi>, "Control Info Cluster out"=w508:T3)  [unwired: 5 in]
                    n145 = Bundle By Name(cluster=w508, "Name"=w507) -> (w502:T3)
                    n146 = call "Add Data Type.vi"("Control Info Cluster in"=w502, "error in (no error)"=w506, "Data Type String"=w503, "Control in"=w505) -> ("error out"=w504:errorcluster, "Control out"=w498:refnum<vi>, "Control Info Cluster out"=w499:T3)  [unwired: 4 in, 1 out]
                    n147 = Build Array (concatenate)(w501, w499) -> (w500:T3[])
                  }
                }
              }
            }
            n148 = Close Reference(reference=w43, error in (no error)=w45) -> (error out=w44:errorcluster)
          }
        }
      }
    }
    frame Error {
    }
  }
  "error out" <- w9
  "Results" <- w3
